vi "Compile - Tx Channel Refs.vi"(6 "Packet Name":string, 7 "Timestamp Present?":bool, 8 "error in (no error)":errorcluster, 11 "Item Ref in":T1 format="%.0x") -> (0 "error out":errorcluster, 2 "Data types":T3[](array[typedef]), 3 "Item Ref out":T1 format="%.0x", 4 "Tx Ref Array":T2 {"VS Refs" format="%.0x"})   [LabVIEW 2016, in "UDP-Custom-Device System Explorer.lvlib"]
uses:
  UDP-Custom-Device System Explorer.lvlib
  Shared/Types/Shared - Channel Data Type.ctl
  <vilib>/NI Veristand/Custom Device API/Custom Device Item Ref.ctl
  Property Accessors/Tx Packet Accessors.lvlib
  <vilib>/NI VeriStand/Custom Device API/Custom Device API.lvlib
  Shared/UDP-Custom-Device Shared.lvlib
  Property Accessors/Shared Packet Accessors.lvlib
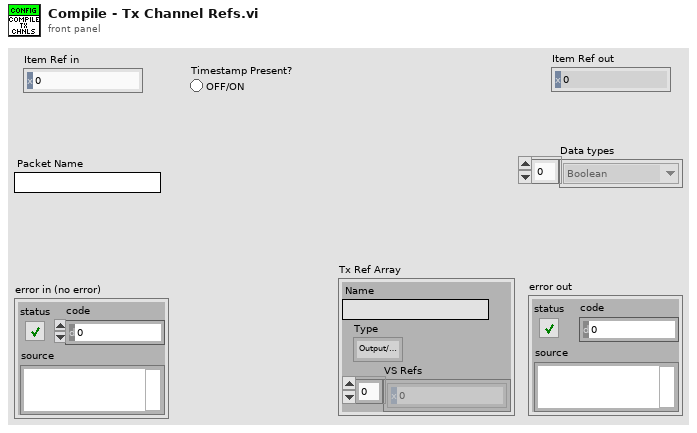
[diagram p1: front panel]
types:
  T1 = typedef "Custom Device API.lvlib/Custom Device Item Ref.ctl" = u64
  T2 = cluster{"Name":string, "Type":enum16{"Output/Write", "Input/Read", "Input/ReadWrite"}, "VS Refs":T1[]}
  T3 = typedef "UDP-Custom-Device Shared.lvlib/Shared - Channel Data Type.ctl" = enum16{"Boolean", "Single", "Double", "I8", "I16", "I32", "I64", "U8", "U16", "U32", "U64"}
  T4 = enum16{"Output/Write", "Input/Read", "Input/ReadWrite"}
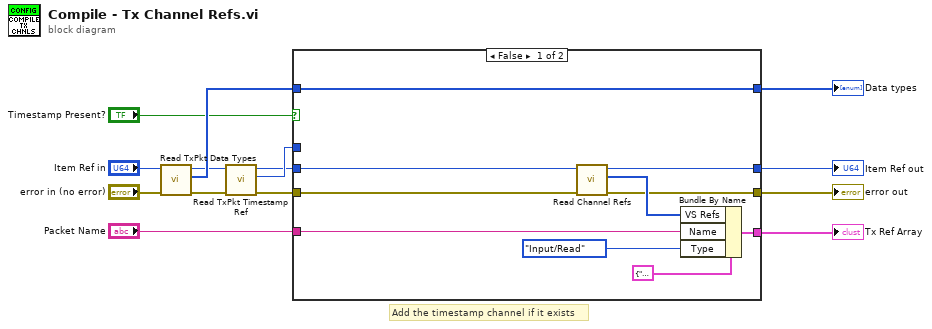
[diagram p0: block diagram]
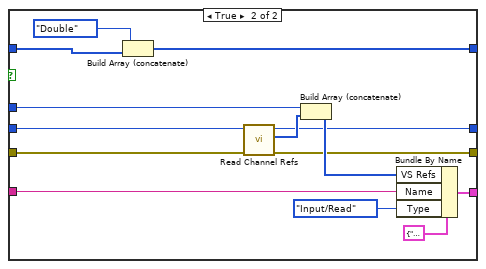
[diagram p2: hidden frame]
diagram:
  # "Add the timestamp channel if it exists"
  n1 = call "Read TxPkt Data Types.vi"("error in (no error)"="error in (no error)", "Node Ptr"="Item Ref in") -> ("error out"=w9:errorcluster, "Data types"=w13:T3[], "Node Ptr out"=w7:T1)  [unwired: 7 in]
  n2 = call "Read TxPkt Timestamp Ref.vi"("error in (no error)"=w9, "Node Ptr"=w7) -> ("error out"=w10:errorcluster, "Timestamp Ref"=w12:T1, "Node Ptr out"=w8:T1)  [unwired: 7 in]
  n3 = case shown="False" "Timestamp Present?" {
    tunnel: [w16 w25] -> w2
    tunnel: "Packet Name" -> [w23 w37]
    tunnel: [w21 w35] -> w4
    tunnel: w8 -> [w19 w29]
    tunnel: w10 -> [w18 w28]
    tunnel: w12 -> [_ w34]
    tunnel: w13 -> [w20 w32]
    tunnel: [w20 w31] -> w14
    tunnel: [w15 w26] -> w1
    frame False {
      n4 = call "Read Channel Refs.vi"("error in (no error)"=w18, "Node Ptr"=w19) -> ("error out"=w16:errorcluster, "Dependent Node Refs"=w17:T1[], "Node Ptr out"=w15:T1)  [unwired: 7 in]
      n5 = Bundle By Name(cluster=T2 {"Name"="", "Type"=enum."Output/Write", "VS Refs"=[]} ("Group"), "VS Refs"=w17, "Name"=w23, "Type"=T4."Input/Read") -> (w21:T2)
    }
    frame True {
      n6 = Build Array (concatenate)(Shared_-_Channel_Data_Type."Double" ("element"), w32) -> (w31:T3[])
      n7 = call "Read Channel Refs.vi"("error in (no error)"=w28, "Node Ptr"=w29) -> ("error out"=w25:errorcluster, "Dependent Node Refs"=w27:T1[], "Node Ptr out"=w26:T1)  [unwired: 7 in]
      n8 = Build Array (concatenate)(w34, w27) -> (w33:T1[])
      n9 = Bundle By Name(cluster=T2 {"Name"="", "Type"=enum."Output/Write", "VS Refs"=[]} ("Group"), "VS Refs"=w33, "Name"=w37, "Type"=T4."Input/Read") -> (w35:T2)
    }
  }
  "Data types" <- w14
  "Tx Ref Array" <- w4
  "error out" <- w2
  "Item Ref out" <- w1
